vi "Configure Output.vi"(7 "Enable Output (T: Enable)":bool=TRUE, 8 "error in (no error)":errorcluster, 9 "Voltage Level (0.0 V)":dbl format="%.3g", 10 "Address (0)":dbl min=0.0 max=31.0 step=1.0 format="%#.0p", 11 "VISA resource name":refnum<visa-resource-name>) -> (0 "error out":errorcluster, 3 "VISA resource name out":refnum<visa-resource-name>)   [LabVIEW 2020, in "BK Precision 911X Series.lvlib"]
doc: "Configures output voltage level and enables or disables the output of the power supply."
uses:
  BK Precision 911X Series.lvlib
panel:
  # "V"
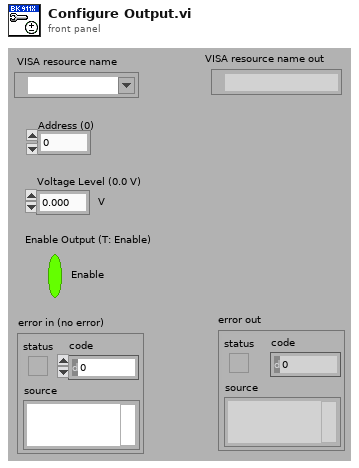
[diagram p1: front panel]
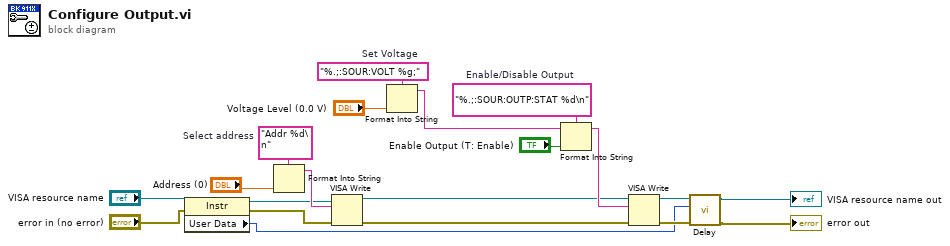
[diagram p0: block diagram]
diagram:
  w17 = "Addr %d\n"  # Select address
  w19 = "%.;:SOUR:OUTP:STAT %d\n"  # Enable/Disable Output
  w20 = "%.;:SOUR:VOLT %g;"  # Set Voltage
  n1 = property class="Instr"(reference="VISA resource name", error in="error in (no error)") -> (reference out=w3:refnum<visa-resource-name>, error out=w2:errorcluster, "User Data"=w1:u32)
  n2 = Format Into String(format string=w17, "Address (0)") -> (resulting string=w16:string)  [unwired: 2 in, 1 out]
  n3 = VISA Write(VISA resource name=w3, write buffer=w16, error in (no error)=w2) -> (VISA resource name out=w11:refnum<visa-resource-name>, error out=w10:errorcluster)  [unwired: 1 out]
  n4 = Format Into String(format string=w20, "Voltage Level (0.0 V)") -> (resulting string=w12:string)  [unwired: 2 in, 1 out]
  n5 = Format Into String(format string=w19, initial string=w12, "Enable Output (T: Enable)") -> (resulting string=w18:string)  [unwired: 1 in, 1 out]
  n6 = VISA Write(VISA resource name=w11, write buffer=w18, error in (no error)=w10) -> (VISA resource name out=w9:refnum<visa-resource-name>, error out=w8:errorcluster)  [unwired: 1 out]
  n7 = call "Delay.vi"("error in (no error)"=w8, "Delay Time (0 ms)"=w1, "VISA resource name"=w9) -> ("error out"=→"error out":errorcluster, "VISA resource name out"=→"VISA resource name out":refnum<visa-resource-name>)  [unwired: 7 in]
